vi "OP500ZP_VG_progressBarOP100ZENplus.vi"() -> ()   [LabVIEW 2020]
panel:
  out "progression":u8(slide) scale=0.0..100.0
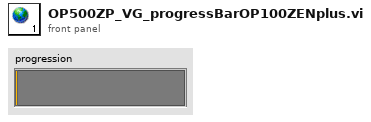
[diagram p1: front panel]
diagram:
